vi "Build Voltage XY Graph Data.vi"(8 "maximum voltage":dbl, 9 "maximum speed":dbl, 10 "cutoff voltage":dbl, 11 "cutoff speed":dbl) -> (3 "XY data":cluster{dbl, dbl}[](array[cluster]))   [LabVIEW 2011, in "Engine Sim System Explorer.lvlib"]
uses:
  Engine Sim System Explorer.lvlib
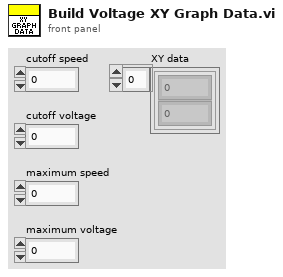
[diagram p1: front panel]
types:
  T1 = cluster{"cutoff speed":dbl, "cutoff voltage":dbl}
  T2 = cluster{"maximum speed":dbl, "maximum voltage":dbl}
  T3 = cluster{"maximum speed":dbl, "maximum voltage":dbl}[]
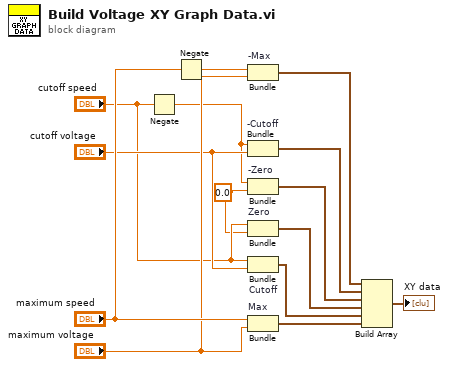
[diagram p0: block diagram]
diagram:
  w4 = 0.0
  n1 = Negate(x="cutoff speed") -> (-x=w6:dbl)
  n2 = Negate(x="maximum speed") -> (-x=w10:dbl)
  n3 = Bundle "-Max"(w10, "maximum voltage"="maximum voltage") -> (w13:cluster{dbl, "maximum voltage":dbl})  [unwired: 1 in]
  n4 = Bundle "-Cutoff"(w6, "cutoff voltage"="cutoff voltage") -> (w7:cluster{dbl, "cutoff voltage":dbl})  [unwired: 1 in]
  n5 = Bundle "-Zero"(w6, w4) -> (w3:cluster{dbl, dbl})  [unwired: 1 in]
  n6 = Bundle "Zero"("cutoff speed"="cutoff speed", w4) -> (w2:cluster{"cutoff speed":dbl, dbl})  [unwired: 1 in]
  n7 = Bundle "Cutoff"("cutoff speed"="cutoff speed", "cutoff voltage"="cutoff voltage") -> (w12:T1)  [unwired: 1 in]
  n8 = Bundle "Max"("maximum speed"="maximum speed", "maximum voltage"="maximum voltage") -> (w14:T2)  [unwired: 1 in]
  n9 = Build Array(w13, w7, w3, w2, w12, w14) -> (→"XY data":T3)
